vi "kąt punktu.vi"(2 "error in":errorcluster, 3 "Pkt":dbl[](array[numeric])) -> (0 "error out":errorcluster, 1 "Kąt":dbl)   [LabVIEW 2016]
doc: "To vi zwraca kąt punktu względem osi OX w przedziale 0 do 2pi"
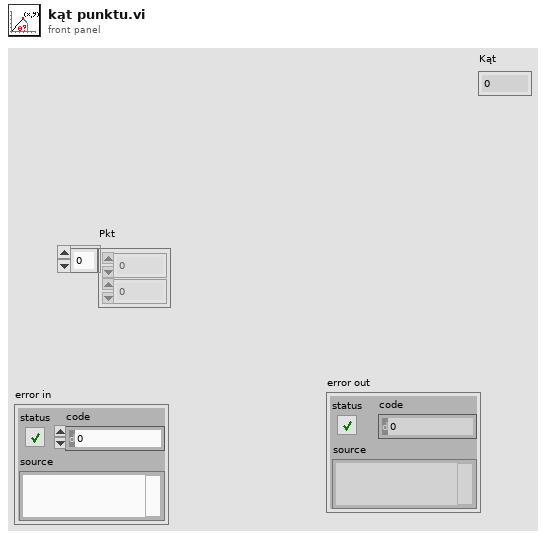
[diagram p1: front panel]
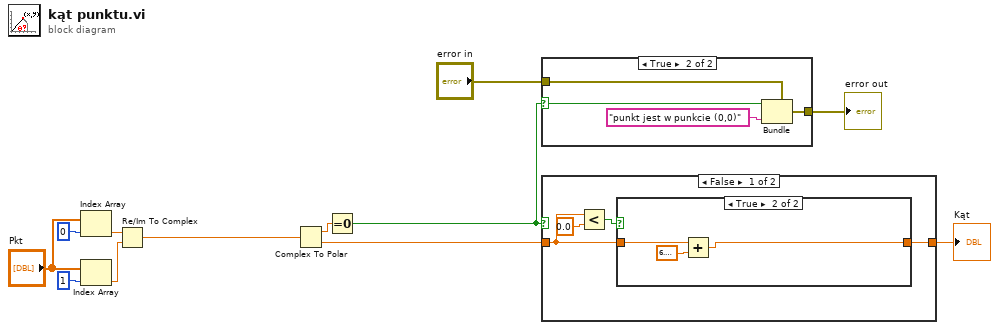
[diagram p0: block diagram]
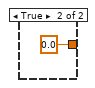
[diagram p3: hidden frame]
diagram:
  n1 = Index Array(array="Pkt", index=0) -> (element=w8:dbl)
  n2 = Index Array(array="Pkt", index=1) -> (element=w7:dbl)
  n3 = Re/Im To Complex(1:w7, 2:w8) -> (0:w6:cdb)
  n4 = Complex To Polar(r * e^(i*theta)=w6) -> (r=w5:dbl, theta=w3:dbl)
  n5 = Equal To 0?(x=w5) -> (x = 0?=w4:bool)
  n6 = case shown="True" w4 {
    selector: w4 -> [_ w16]
    tunnel: "error in" -> [w13 w17]
    tunnel: [w13 w14] -> w2
    frame False {
    }
    frame True {
      n7 = Bundle(cluster=w17, "status"=w16, "source"="punkt jest w punkcie (0,0)") -> (w14:errorcluster)  [unwired: 1 in]
    }
  }
  "error out" <- w2
  n8 = case shown="False" w4 {
    tunnel: w3 -> [w19 _]
    tunnel: [w18 0.0] -> w1
    frame False {
      n9 = Less?(x=w19, y=0.0) -> (x < y?=w20:bool)
      n10 = case shown="True" w20 {
        tunnel: w19 -> [w22 w25]
        tunnel: [w22 w23] -> w18
        frame False {
        }
        frame True {
          n11 = Add(x=w25, y=6.283185307179586) -> (x+y=w23:dbl)
        }
      }
    }
    frame True {
    }
  }
  "Kąt" <- w1
